vi "Test Append Row Values.vi"(11 "Test Case In":refnum<class "Test Open Xml.lvclass">) -> (0 "error out":errorcluster, 3 "Test Case Out":refnum<class "Test Open Xml.lvclass">)   [LabVIEW 2020, in "Test Open Xml.lvclass"]
uses:
  Test Open Xml.lvclass
  C:/Program Files/National Instruments/LabVIEW 2025/vi.lib/Astemes/LUnit/Test Case.lvclass
  Source/Cell DataType.ctl
  <vilib>/Astemes/LUnit/Test Case.lvclass/Test Case.ctl
  a710e01d-083e-4ad4-93ae-fbf4f3e7ce4d.vi
  e5169541-515f-4f16-96fe-0f2d3de234a9.vi
  <vilib>/Astemes/LUnit/Core/LUnit Test Case/Private/Append Fail Result.vi
  <vilib>/Astemes/LUnit/Core/LUnit Test Case/Private/Append Pass Result.vi
  <vilib>/Astemes/LUnit/Core/LUnit Test Case/Private/Run In UI.vi
  <vilib>/Utility/error.llb/Clear Errors.vi
  <vilib>/Astemes/LUnit/Test Case.lvclass
  Source/Open Xml.lvlib
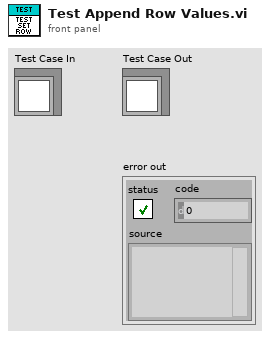
[diagram p1: front panel]
types:
  T1 = typedef "Open Xml.lvlib/Cell DataType.ctl" = enum16{"Void", "Boolean", "Number", "Error", "SharedString", "String", "InlineString", "Date"}
  T2 = cluster{"Number":dbl, "String":string, "Boolean":bool, "Time Stamp":timestamp, "Error":errorcluster}[]
  T3 = cluster{"Number":dbl, "String":string, "Boolean":bool, "Time Stamp":timestamp, "Error":errorcluster}
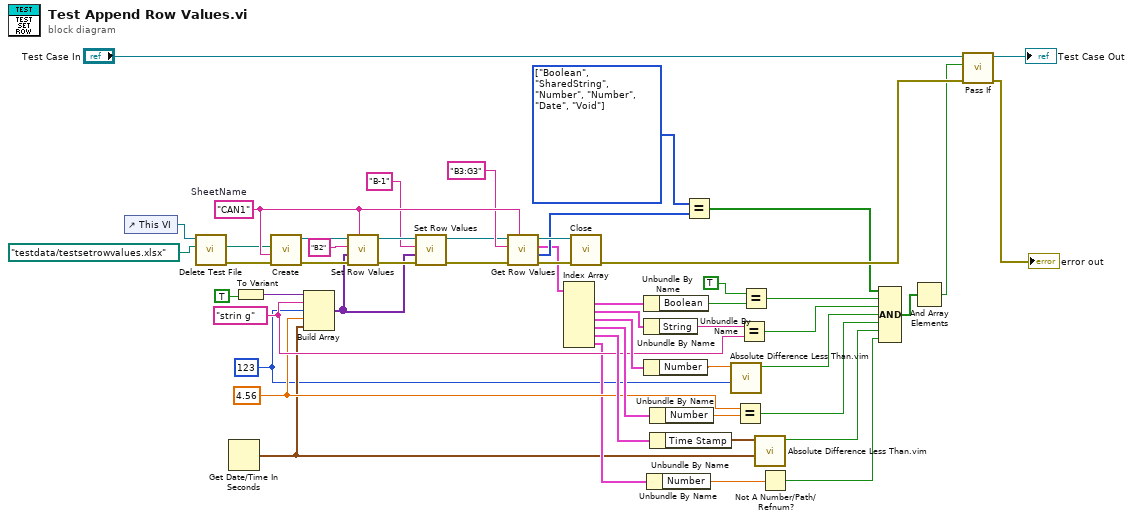
[diagram p0: block diagram]
diagram:
  w34 = T1[] [enum."Boolean", enum."SharedString", enum."Number", enum."Number", enum."Date", enum."Void"] items=["Void", "Boolean", "Number", "Error", "SharedString", "String", "InlineString", "Date"] ("x")
  w18 = 4.56
  w6 = 123
  w20 = "strin g"
  w44 = "CAN1"  # SheetName
  n1 = control-ref of="This VI"() -> (w11:refnum<vi>)
  n2 = call "Delete Test File.vi"("name or relative path"=path "testdata/testsetrowvalues.xlsx", "VI in"=w11) -> ("error out"=w12:errorcluster, "deleted path"=w9:path)  [unwired: 8 in]
  n3 = Get Date/Time In Seconds() -> (seconds since 1Jan1904=w7:timestamp)
  n4 = To Variant(anything=TRUE) -> (Variant=w38:variant)
  n5 = call "Create.vi"("error in"=w12, "SheetName"=w44, "Path"=w9) -> ("error out"=w48:errorcluster, "SpreadsheetDoc"=w49:refnum<k24>)  [unwired: 7 in]
  n6 = Build Array(w38, w20, w6, w18, w7) -> (w1:variant[])
  n7 = call "Set Row Values.vi"("Sheet Name"=w44, "error in"=w48, "Values"=w1, "Cell Address"="B2", "SpreadsheetDoc"=w49) -> ("error out"=w42:errorcluster, "SpreadsheetDoc out"=w4:refnum<k24>)  [unwired: 5 in]
  n8 = call "Set Row Values.vi"("error in"=w42, "Values"=w1, "Cell Address"="B-1", "SpreadsheetDoc"=w4) -> ("error out"=w5:errorcluster, "SpreadsheetDoc out"=w3:refnum<k24>)  [unwired: 6 in]
  n9 = call "Get Row Values.vi"("Sheet Name"=w44, "error in"=w5, "Row Address"="B3:G3" ("Cell Address"), "SpreadsheetDoc in"=w3) -> ("error out"=w46:errorcluster, "Types"=w41:T1[], "Cell Values"=w35:T2, "SpreadsheetDoc out"=w45:refnum<k24>)  [unwired: 4 in]
  n10 = Index Array(array=w35) -> (element #1=w33:T3, element #2=w32:T3, element #3=w31:T3, element #4=w30:T3, element #5=w29:T3, element #6=w15:T3)  [unwired: 6 in]
  n11 = call "Close.vi"("error in"=w46, "SpreadsheetDoc"=w45) -> ("error out"=w47:errorcluster)  [unwired: 9 in]
  n12 = Unbundle By Name(w33) -> ("Boolean"=w25:bool)
  n13 = Unbundle By Name(w32) -> ("String"=w22:string)
  n14 = Unbundle By Name(w31) -> ("Number"=w27:dbl)
  n15 = Unbundle By Name(w15) -> ("Number"=w13:dbl)
  n16 = Unbundle By Name(w30) -> ("Number"=w19:dbl)
  n17 = Unbundle By Name(w29) -> ("Time Stamp"=w26:timestamp)
  n18 = Equal?(x=w34, y=w41) -> (x = y?=w40:bool[])
  n19 = call "Absolute Difference Less Than.vim"("Number 2"=w6, "Number 1"=w27) -> ("In Limit"=w8:bool)  [unwired: 9 in]
  n20 = Equal?(x=w18, y=w19) -> (x = y?=w17:bool)
  n21 = Equal?(x=w22, y=w20) -> (x = y?=w21:bool)
  n22 = Equal?(x=TRUE, y=w25) -> (x = y?=w23:bool)
  n23 = call "Absolute Difference Less Than.vim"("Number 2"=w7, "Number 1"=w26) -> ("In Limit"=w16:bool)  [unwired: 9 in]
  n24 = Not A Number/Path/Refnum?(number/path/refnum=w13) -> (NaN/Path/Refnum?=w14:bool)
  n25 = Compound Arithmetic op=AND(w40, w23, w21, w8, w17, w16, w14) -> (w28:bool[])
  n26 = And Array Elements(Boolean array=w28) -> (logical AND=w43:bool)
  n27 = call <vilib>:"Pass If.vi"("error in (no error)"=w47, "Pass?"=w43, "LUnit Test Case In"="Test Case In") -> ("error out"=→"error out":errorcluster, "LUnit Test Case Out"=→"Test Case Out":refnum<class "Test Open Xml.lvclass">)  [unwired: 7 in]
